vi "test_Create Periodic & Trigger Message.vi"(8 "error in (no error)":errorcluster, 11 "TestCase in":refnum<class "Instrument Addon Scripting API Messages Unit Tests.lvclass">) -> (0 "error out":errorcluster, 3 "TestCase out":refnum<class "Instrument Addon Scripting API Messages Unit Tests.lvclass">)   [LabVIEW 2018, in "Instrument Addon Scripting API Messages Unit Tests.lvclass"]
uses:
  Instrument Addon Scripting API Messages Unit Tests.lvclass
  Addon/Addon Shared/Types/Message Generation Type.ctl
  Addon/Addon Shared/Types/FG Control.ctl
  NationalInstruments.VeriStand.SystemDefinitionAPI
  APIs/Scripting API/TypeDefs/Message Settings.ctl
  APIs/Scripting API/TypeDefs/Protection Types.ctl
  Addon/Addon Shared/SubVIs/Constants.vi
  <vilib>/NI Veristand/Custom Device Tools/Custom Device Utility Library/NI VeriStand - Search for Item by GUID.vi
  APIs/Scripting API/Messages/Create Message - Periodic & Trigger.vi
  <vilib>/NI Veristand/Custom Device API/NI VeriStand - Get Item Property.vi
  <vilib>/NI Veristand/Custom Device API/Get Item Property (Boolean).vi
  <vilib>/NI Veristand/Custom Device API/Get Item Property (String).vi
  <vilib>/NI Veristand/Custom Device API/NI VeriStand - Set Item Property.vi
  <vilib>/NI Veristand/Custom Device API/Set Item Property (Boolean).vi
  <vilib>/NI Veristand/Custom Device API/Set Item Property (String).vi
  <vilib>/NI Veristand/Custom Device API/Get Item Property (U32).vi
  <vilib>/NI Veristand/Custom Device API/Get Item Property (Double).vi
  <vilib>/NI Veristand/Custom Device API/Set Item Property (U32).vi
  <vilib>/NI Veristand/Custom Device API/Set Item Property (Double).vi
  <vilib>/addons/_JKI Toolkits/VI Tester/TestCase.llb/TestCase.lvclass
  Instrument Addon Scripting API Test Assets/Instrument Addon Scripting API Test Assets.lvclass
  APIs/Scripting API/Instrument Addon Scripting API.lvlib
  <vilib>/NI Veristand/Custom Device Tools/Custom Device Utility Library/Custom Device Utility Library.lvlib
  Addon/Addon Shared/Instrument Addon Shared.lvlib
  C:/Program Files (x86)/National Instruments/LabVIEW 2018/vi.lib/addons/_JKI Toolkits/VI Tester/TestCase.llb/TestCase.lvclass
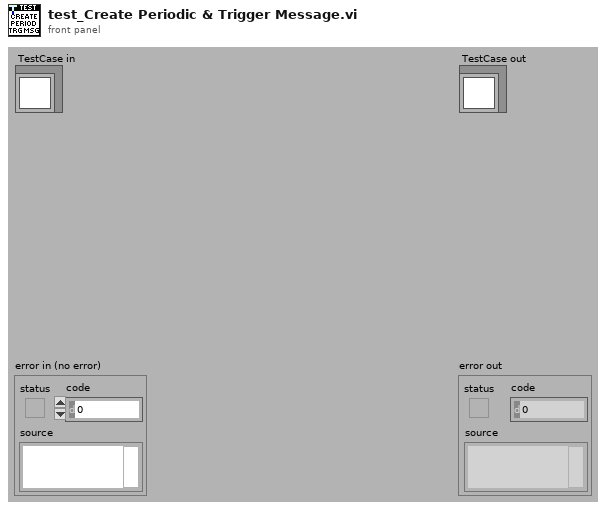
[diagram p1: front panel]
types:
  T1 = typedef "Instrument Addon Shared.lvlib/FG Control.ctl" = enum16{"Get", "Set"}
  T2 = typedef "Instrument Addon Shared.lvlib/Message Generation Type.ctl" = enum16{"Trigger Only", "Periodic & Trigger", "Value Change & Trigger"}
  T3 = typedef "Instrument Addon Scripting API.lvlib/Message Settings.ctl" = cluster{"Protection Types":T4, "Enable Periodic Default":bool, "Trigger Channel Refnum":u64}
  T4 = typedef "Instrument Addon Scripting API.lvlib/Protection Types.ctl" = enum16{"None", "CRC-32", "Checksum U16", "Checksum U32", "Checksum U8"}
  T5 = typedef "Custom Device API.lvlib/Custom Device Item Ref.ctl" = u64
  T6 = typedef "Instrument Addon Shared.lvlib/Trigger Parameters.ctl" = cluster{"Use Channel":bool, "Channel Path":string}
  T7 = typedef "Instrument Addon Shared.lvlib/Message Parameters.ctl" = cluster{"Generation Type":T2, "Period":dbl, "Include Protection":bool, "Type":string}
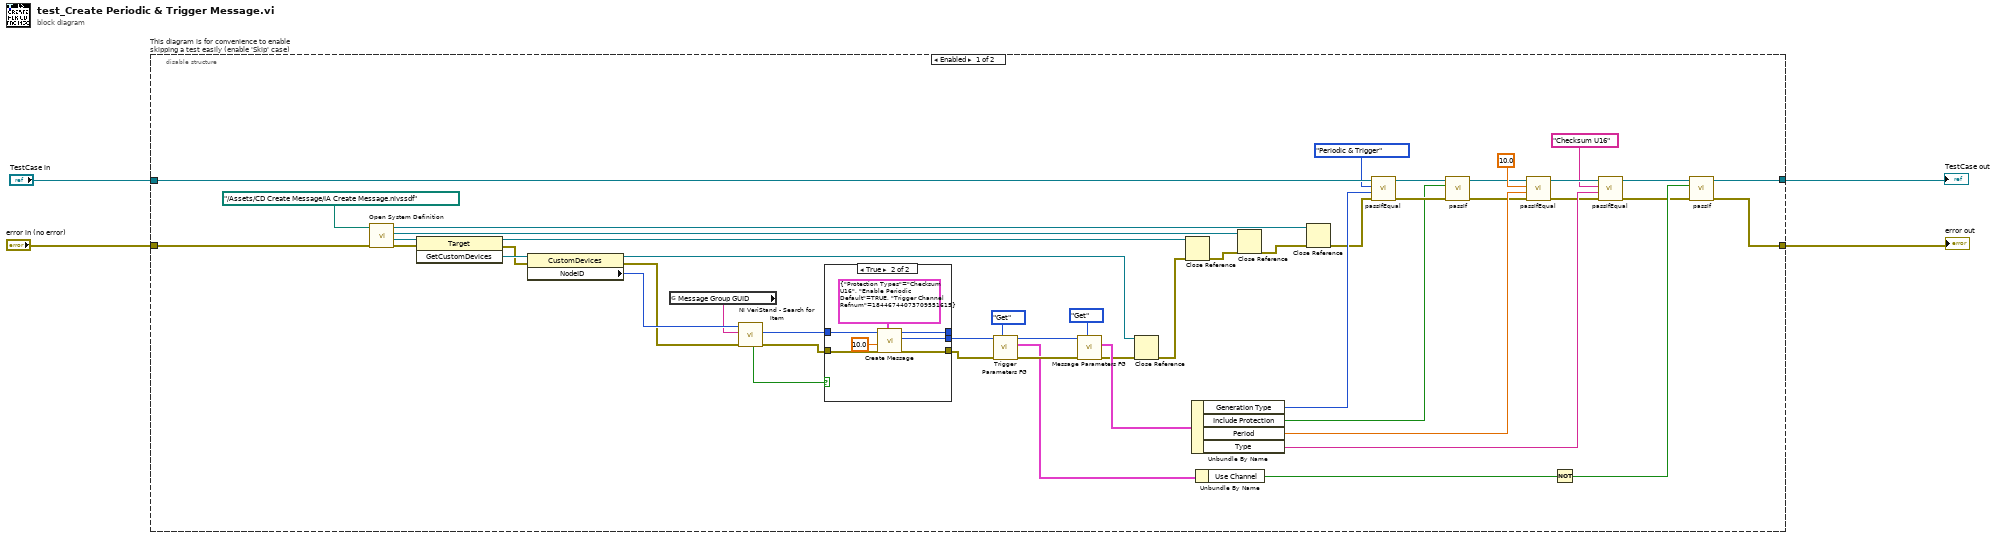
[diagram p0: block diagram]
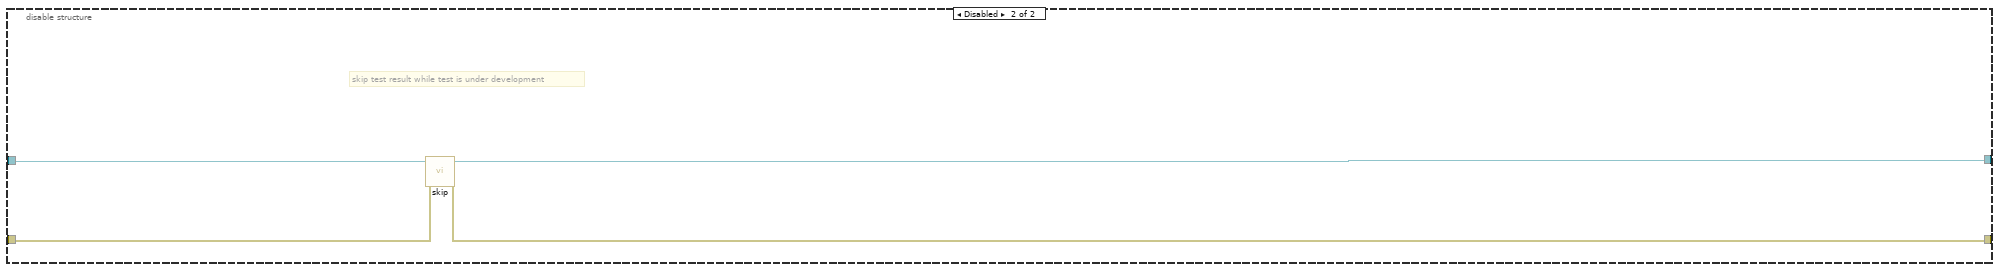
[diagram p3: hidden frame]
diagram:
  n1 = disable-structure "This diagram is for convenience to enable skipping a test easily (enable 'Skip' case)" shown="Enabled" {
    disable-tunnel: "TestCase in" -> [w37 w65]
    disable-tunnel: [w15 w63] -> w1
    disable-tunnel: [w16 w64] -> w3
    disable-tunnel: "error in (no error)" -> [w52 w62]
    frame Enabled {
      n2 = call "Open System Definition.vi"("error in (no error)"=w52, "System Definition File"=path "../Assets/CD Create Message/IA Create Message.nivssdf" ("SDF file")) -> ("error out"=w45:errorcluster, "Target Refnum"=w51:refnum<k24>, "Root Refnum"=w40:refnum<k24>, "System Definition Refnum"=w14:refnum<k24>)  [unwired: 6 in]
      n3 = invoke class="Target" method="GetCustomDevices"(reference=w51, error in=w45) -> (reference out=w7:refnum<k24>, error out=w44:errorcluster, "GetCustomDevices"=w50:refnum<k24>)  [unwired: 1 in]
      n4 = property class="CustomDevices"(reference=w50, error in=w44) -> (reference out=w41:refnum<k24>, error out=w43:errorcluster, "NodeID"=w49:u64)
      n5 = global read "Constants.vi" "Message Group GUID"() -> (w48:string)
      n6 = call-poly <vilib>:"NI VeriStand - Search for Item.vi"("error in"=w43, "Item GUID"=w48, "Section Ref in"=w49) -> ("error out"=w42:errorcluster, "Item Ref"=w47:T5, "Found"=w46:bool)  [unwired: 5 in, 1 out]
      n7 = case shown="True" w46 {
        tunnel: w47 -> [_ w61]
        tunnel: [w54 w60] -> w25
        tunnel: w42 -> [w54 w59]
        tunnel: [_ w58] -> w23
        tunnel: [_ w57] -> _
        frame False {
        }
        frame True {
          n8 = call-poly "Create Message.vi"("Message Settings"=T3 {"Protection Types"=enum."Checksum U16", "Enable Periodic Default"=TRUE, "Trigger Channel Refnum"=18446744073709551615}, "error in (no error)"=w59, "Period (s)"=10.0 ("Period"), "Message Group in"=w61) -> ("error out"=w60:errorcluster, "Message Refnum out"=w58:T5, "Message Goup out"=w57:T5)  [unwired: 5 in]
        }
      }
      n9 = call "Trigger Parameters FG.vi"("Action"=FG_Control."Get", "error in (no error)"=w25, "Item Ref in"=w23) -> ("error out"=w24:errorcluster, "Trigger Parameters"=w21:T6, "Item Ref out"=w22:T5)  [unwired: 6 in]
      n10 = call "Message Parameters FG.vi"("Action"=FG_Control."Get", "error in (no error)"=w24, "Item Ref in"=w22) -> ("error out"=w34:errorcluster, "Message Settings out"=w38:T7)  [unwired: 6 in, 1 out]
      n11 = Close Reference(reference=w41, error in (no error)=w34) -> (error out=w6:errorcluster)
      n12 = Close Reference(reference=w7, error in (no error)=w6) -> (error out=w5:errorcluster)
      n13 = Unbundle By Name(w38) -> ("Generation Type"=w36:T2, "Include Protection"=w8:bool, "Period"=w32:dbl, "Type"=w29:string)
      n14 = Unbundle By Name(w21) -> ("Use Channel"=w20:bool)
      n15 = Close Reference(reference=w40, error in (no error)=w5) -> (error out=w13:errorcluster)
      n16 = Close Reference(reference=w14, error in (no error)=w13) -> (error out=w33:errorcluster)
      n17 = call-dynamic "passIfEqual.vi"("error in (no error)"=w33, "y"=w36, "x"=Message_Generation_Type."Periodic & Trigger" ("Generation Type"), "TestCase in"=w37) -> ("error out"=w12:errorcluster, "TestCase out"=w10:refnum<class "Instrument Addon Scripting API Messages Unit Tests.lvclass">)  [unwired: 6 in]
      n18 = call-dynamic "passIf.vi"("error in (no error)"=w12, "pass"=w8, "TestCase in"=w10) -> ("error out"=w11:errorcluster, "TestCase out"=w9:refnum<class "Instrument Addon Scripting API Messages Unit Tests.lvclass">)  [unwired: 7 in]
      n19 = call-dynamic "passIfEqual.vi"("error in (no error)"=w11, "y"=w32, "x"=10.0 ("Period"), "TestCase in"=w9) -> ("error out"=w27:errorcluster, "TestCase out"=w30:refnum<class "Instrument Addon Scripting API Messages Unit Tests.lvclass">)  [unwired: 6 in]
      n20 = Not(x=w20) -> (.not. x?=w19:bool)
      n21 = call-dynamic "passIfEqual.vi"("error in (no error)"=w27, "y"=w29, "x"="Checksum U16" ("Type"), "TestCase in"=w30) -> ("error out"=w18:errorcluster, "TestCase out"=w17:refnum<class "Instrument Addon Scripting API Messages Unit Tests.lvclass">)  [unwired: 6 in]
      n22 = call-dynamic "passIf.vi"("error in (no error)"=w18, "pass"=w19, "TestCase in"=w17) -> ("error out"=w16:errorcluster, "TestCase out"=w15:refnum<class "Instrument Addon Scripting API Messages Unit Tests.lvclass">)  [unwired: 7 in]
    }
    frame Disabled {
      # "skip test result while test is under development"
      n23 = call <vilib>:"skip.vi"("error in (no error)"=w62, "TestCase in"=w65) -> ("error out"=w64:errorcluster, "TestCase out"=w63:refnum<class "Instrument Addon Scripting API Messages Unit Tests.lvclass">)  [unwired: 8 in]
    }
  }
  "error out" <- w3
  "TestCase out" <- w1
